vi "Read Attributes.vi"(11 "Stop Microgrid Msg":refnum<class "Stop Microgrid Msg.lvclass">) -> (2 "Payload":cluster{"Variant":variant})   [LabVIEW 2018, in "Remote Operation Abstract.lvlib" / "Stop Microgrid Msg.lvclass"]
uses:
  Stop Microgrid Msg.lvclass
  Stop Microgrid Msg.lvclass/Stop Microgrid Msg.ctl
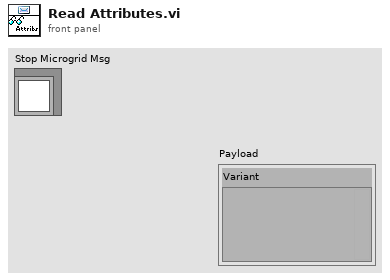
[diagram p1: front panel]
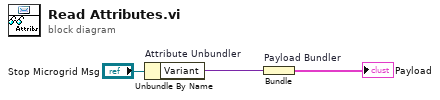
[diagram p0: block diagram]
diagram:
  n1 = Unbundle By Name "Attribute Unbundler"("Stop Microgrid Msg") -> ("Variant"=w1:variant)
  n2 = Bundle "Payload Bundler"("Variant"=w1) -> (→"Payload":cluster{"Variant":variant})  [unwired: 1 in]
